vi "Machine Cal UI.vi"() -> ()   [LabVIEW 2013]
uses:
  <vilib>/ptbypt/NI_PtbyPt.lvlib
  <vilib>/Utility/miscctls.llb/LVRowAndColumnTypeDef.ctl
  <vilib>/Analysis/NI_AALPro.lvlib
  Type Defs/Registered Machines.ctl
  <vilib>/Utility/file.llb/Read From Spreadsheet File (string).vi
  <vilib>/event_ctls.llb/lveventtype.ctl
panel:
  in  "View Spreadsheet":bool
  in  "Cal Certificate Path":path
  in  "Cal Cert Started":bool
  in  "Tab.Screen":T1(tab)
  in  "Connection Error":T2(tab)
  in  "Action to Perform":u16(ring) items=["", "Start Calibration", "Continue Calibration", "System Initialization", "System Closeout"]
  in  "IP 4":u8
  in  "IP 3":u8
  in  "IP 2":u8
  in  "IP 1":u8 caption="IP Address"
  in  "pb.sys_connect":bool
  in  "System Type":u16(ring) items=["Continuous Monitoring Tank", "Continuous Module Tank", "Standard Gas Rack", "High-Flow Gas Rack", "Warranty Gas Rack", "Hot Fuel Chamber"]
  in  "Calibration Details":string[][](table)
  in  "Instrument Identification":string[][](table)
  in  "Environment Details":string[][](table)=[["TI Automotive"], ["Caro Test Center"], ["628 Columbia St."], ["Caro, MI 48723"]]
  in  "Standards Used":string[][](table)
  in  "pb.ChanSetup_Forward":bool
  in  "pb.Quit Cal":bool
  in  "Channel Descriptions:":string[][](table)
  in  "Machine Specifications:":string[][](table)
  in  "pb.InfoPage_Back":bool
  in  "pb.SelectionPage_Forward":bool
  in  "pb.ChanSetup_Back":bool
  in  "pb.Cal/Ver_Forward":bool
  in  "Select Units:":enum16{""}(ring)
  out "Tracking":string[][](table)
  in  "Channels Selected:":i32
  in  "pb.Coefficients":bool
  in  "Temperature of room (C)":dbl
  in  "Relative Humidity (%)":dbl
  out "State:":string
  in  "pb.Activate Channels":bool
  in  "Checkbox 12":bool
  in  "pb.Apply 5":bool
  in  "pb.Apply 4":bool
  in  "pb.Apply 3":bool
  in  "pb.Apply 2":bool
  in  "Master Reading":dbl
  in  "Checkbox 2":bool
  in  "Checkbox 1":bool
  out "Units":string
  out "Unit Abbreviation":string
  in  "Channels":string[][](table)=[["", "", "", "", "", "", "", "", "", "", ""]]
  in  "Readings":dbl[](array[numeric])
  in  "pb.Apply 1":bool
  in  "Checkbox 3":bool
  in  "Checkbox 4":bool
  in  "Checkbox 5":bool
  in  "Checkbox 6":bool
  in  "Checkbox 7":bool
  in  "Checkbox 8":bool
  in  "Checkbox 9":bool
  in  "Checkbox 10":bool
  in  "Checkbox 11":bool
  in  "pb.SelectionPage_Back":bool
  in  "[Checkboxes]":T3
  # "*Excel must be closed to return control to this app."
  # "Former Pane: H=499  W=1030"
  # "Tab: H=495  W=1026"
  # "Now thinking it would be better to\nstore that on the RIOs"
  # "Need to have a way to differentiate between a\nnew cal and continuing a cal that is in process"
  # "IP Address"
  # "New System\nCal existing system\nSystem Closeout"
  # "*"
  # "*"
  # "System Not Registered"
  # "*"
  # "*"
  # "*"
  # "*"
  # "System Connection Issue"
  # "*"
  # "*"
  # "*"
  # "*"
  # "RIO Import Issue"
  # "*"
  # "*"
  # "Cannot allow duplicate unit abbreviations or what standard is used to calibrate\na channel is not documented"
  # "Was going to just use a cursive\nfont but dont know if that would\nconstitute a true electronic\nsignature and was not finding\nclear definitions with a quick search"
  # "should be programmatically handled with dropdowns..."
  # "Was thinking I would put expected cal and verify points but I think that\nmight be a problem when it comes to the option of doing multiple\nchannels at once and maybe 1 position used a different cal point"
  # "programmed to the unit abbreviations from channel setup machine specifications"
  # "abbr."
  # "Should always display all and highlight first 4 columns of selected rows"
  # "...have not thought through getting new coefficients would happen"
  # "Incomplete---------------------------------Green\nDone                                                                  Red"
  # "As found\nCalibrate\nVerify"
  # "When I take/retake all readings prompt that new\ncoefficients exist would you like to apply\n\nwould then need a way to store those in case\nthey do not want to apply immediately"
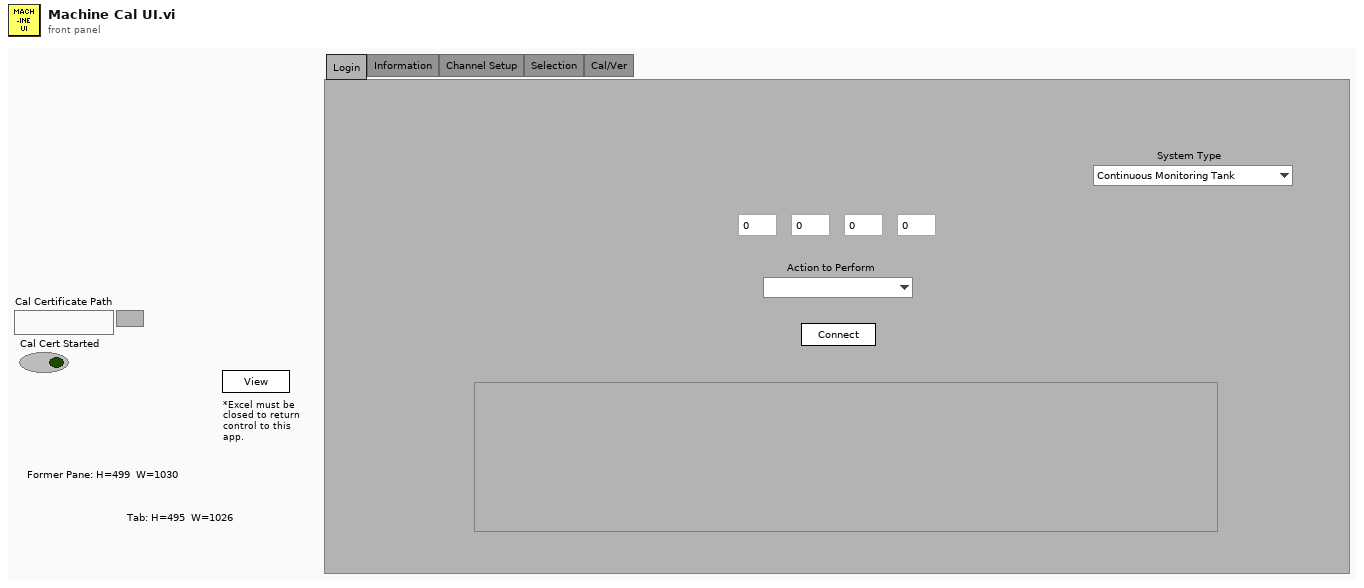
[diagram p1: front panel]
types:
  T1 = enum32{"Login", "Information", "Channel Setup", "Selection", "Cal/Ver"}
  T2 = enum32{"Registration", "Connection", "RIO Import"}
  T3 = cluster{"CB1":bool, "CB2":bool, "CB3":bool, "CB4":bool, "CB5":bool, "CB6":bool, "CB7":bool, "CB8":bool, "CB9":bool, "CB10":bool, "CB11":bool, "CB12":bool}
  T4 = typedef "Registered Machines.ctl" = cluster{"Serial Number":string, "ID":string}
  T5 = cluster{"Certificate Template":path, "Cal Certificate Path":path, "Cal Cert Started":bool, "CalType":u16, "Registered Systems":T4[], "Cal Files Path":path, "Environment Details":string[][], "Instrument Identification":string[][], "Standards Used":string[][], "Calibration Details":string[][], "Machine Specifications:":string[][], "Channel Descriptions:":string[][], "Tracking":string[][], "TrackingRowsSel":i32[], "TrackingTableColors":i32[][], "CalChannelsStorage":string[][], "CalChannelsDisplay":string[][], "ServerStorageFolder":path, "Date FolderPath":path, "Page":enum32{"Login", "Information", "Channel Setup", "Selection", "Cal/Ver"}, "Scroll Flag":bool, "Scroll Check":bool, "Channel Offset":i32, "Checkbox Array":bool[], "Read Array":bool[], "Data Active":bool, "Data Timer":dbl, "Data Timing":dbl, "Full Data":dbl[], "MasterCol":i32, "MasterReading":dbl, "Cal/Ver Data":dbl[], "RIOprogram":string, "IPstring":string, "RIOTempFolder":path, "ServerTempFolder":path, "RoomTemp":dbl, "RelHumidity":dbl, "MaskReadings":bool, "CalState":string, "FoundChannelsStorage":string[][], "VerChannelsStorage":string[][]}
  T6 = enum8{"Enabled", "Disabled", "Disabled and Grayed Out"}
  T7 = enum16{"Init", "Start Data", "Stop Data", "Lost Connection", "Engine Idle", "Write Data", "Read Data"}
  T8 = typedef "lveventtype.ctl" = enum32{"Null", "Timeout", "Annotation Menu Selection", "Annotation Menu Selection?", "App Instance Close", "App Instance Close?", "Autoscale Range Change", "Bookmark Info Change", "Cell Edit", "Cell Edit?", "Cursor Grab", "Cursor Grab?", "Cursor Menu Selection", "Cursor Menu Selection?", "Cursor Move", "Cursor Release", "Data Change", "Direction Change", "Display State Change", "Drag Ended", "Drag Enter", "Drag Leave", "Drag Over", "Drag Source Update", "Drag Starting", "Drag Starting?", "Drop", "Exec State Change", "Key Down", "Key Down?", "Key Repeat", "Key Repeat?", "Key Up", "Listbox Double Click", "Menu Activation?", "Menu Selection (App)", "Menu Selection? (App)", "Menu Selection (User)", "Mouse Down", "Mouse Down?", "Mouse Enter", "Mouse Leave", "Mouse Move", "Mouse Up", "Mouse Wheel", "NI Security User Change (App)", "Pane Size", "Panel Close", "Panel Close?", "Panel Resize", "Plot Attribute Change", "Scale Range Change", "Shortcut Menu Activation?", "Shortcut Menu Selection (App)", "Shortcut Menu Selection? (App)", "Shortcut Menu Selection (User)", "Tree Double Click", "Tree Drag", "Tree Drag?", "Tree Drop", "Tree Drop?", "Tree Item Close", "Tree Item Close?", "Tree Item Open", "Tree Item Open?", "User Event", "Value Change"}
  T9 = typedef "LVRowAndColumnTypeDef.ctl" = cluster{"Row":i32, "Column":i32}
  T10 = typedef "eventvkey.ctl" = enum16{"ASCII", "Enter", "Return", "Shift", "Ctrl", "Alt", "Cmd", "Opt", "Caps", "NumLock", "Clear", "Break", "Up", "Down", "Left", "Right", "Insert", "Delete", "Home", "End", "PageUp", "PageDown", "Escape", "Help", "Pause", "ScrollLock", "F1", "F2", "F3", "F4", "F5", "F6", "F7", "F8", "F9", "F10", "F11", "F12", "F13", "F14", "F15", "F16", "F17", "F18", "F19", "F20", "F21", "F22", "F23", "F24", "Play", "VolumeUp", "VolumeDown", "Mute", "Two Byte Char"}
  T11 = typedef "LVPoint32TypeDef.ctl" = cluster{"Horizontal":i32, "Vertical":i32}
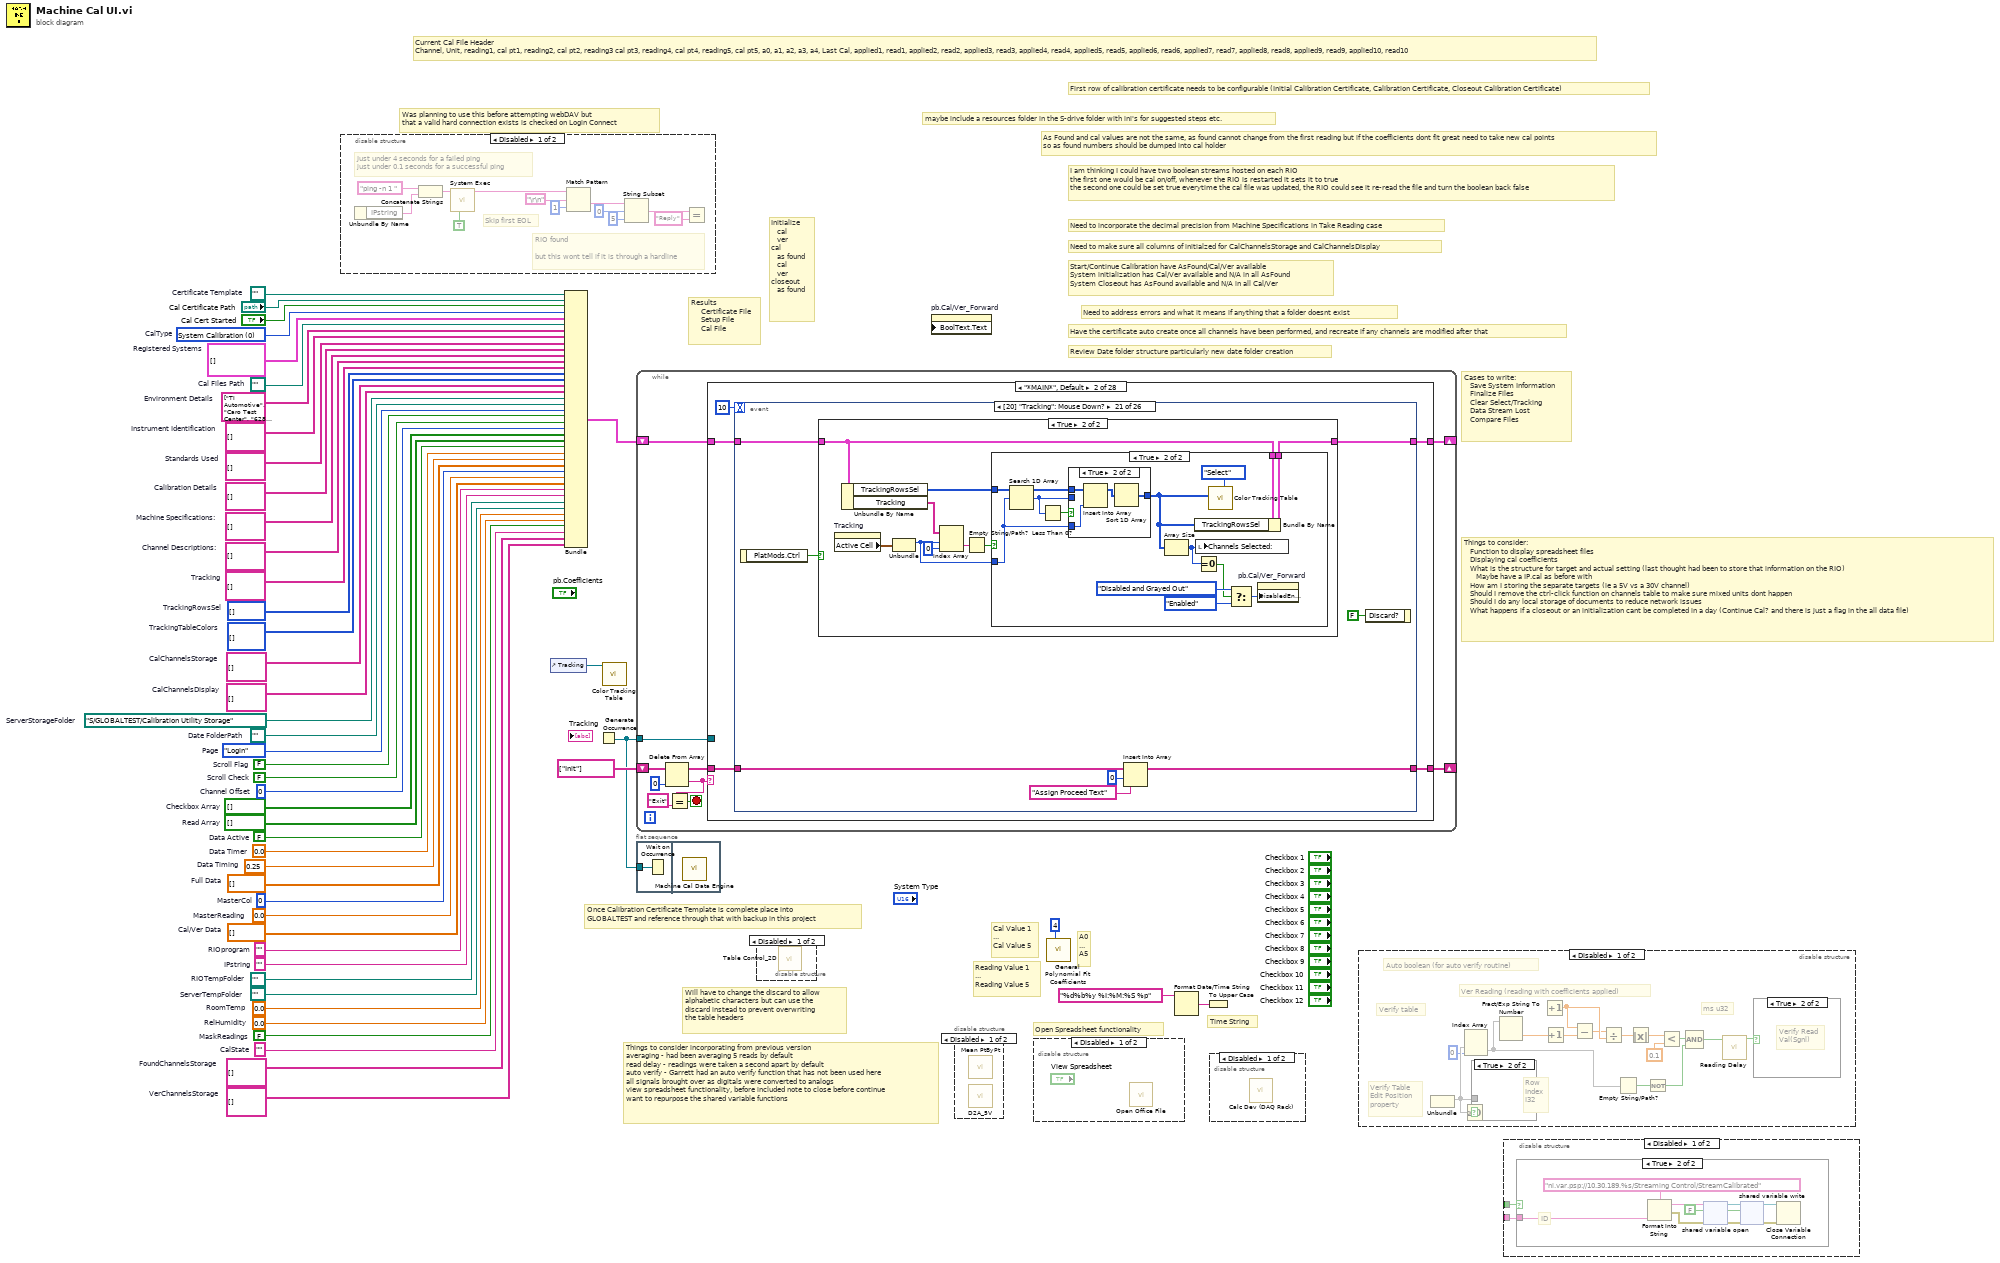
[diagram p0: block diagram]
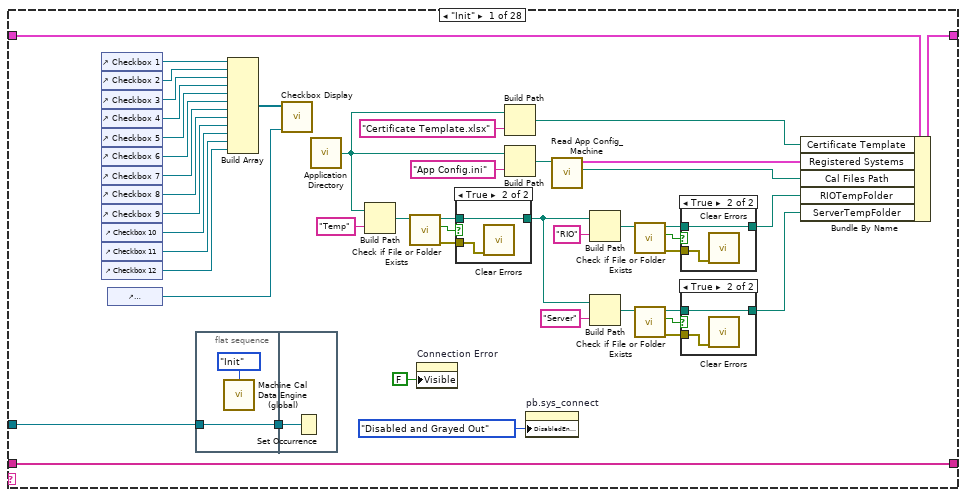
[diagram p12: hidden frame]
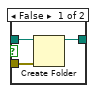
[diagram p13: hidden frame]
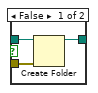
[diagram p14: hidden frame]
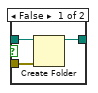
[diagram p15: hidden frame]
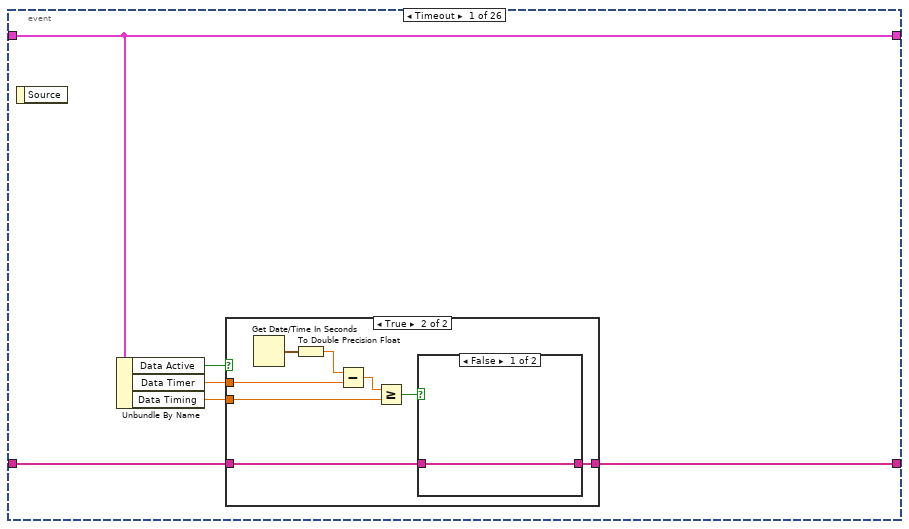
[diagram p16: hidden frame]
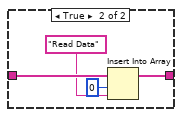
[diagram p18: hidden frame]
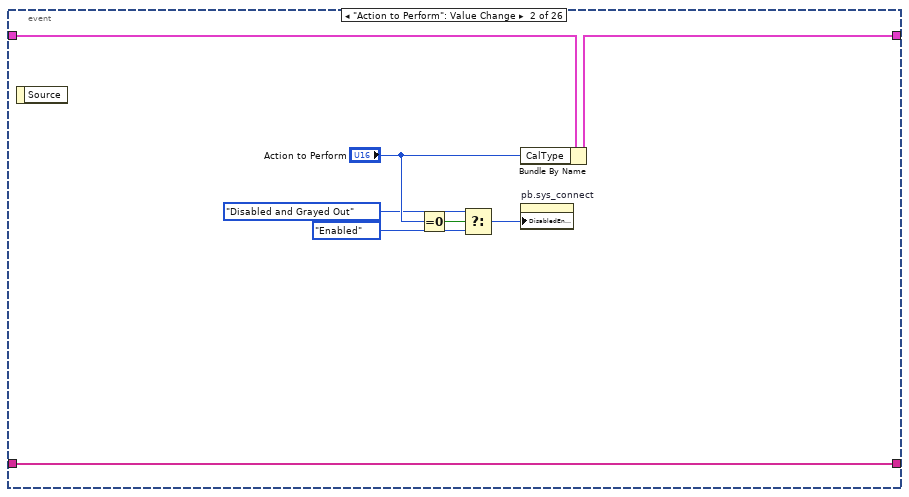
[diagram p19: hidden frame]
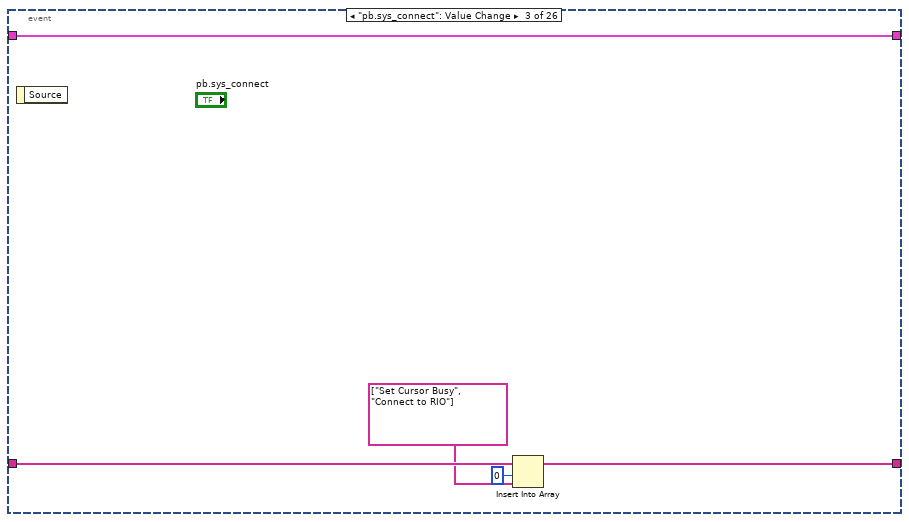
[diagram p20: hidden frame]
diagram:
  w1 = string[][] []  # VerChannelsStorage
  w2 = string[][] []  # FoundChannelsStorage
  w3 = ""  # CalState
  w7 = FALSE  # MaskReadings
  w8 = 0.0  # RelHumidity
  w9 = 0.0  # RoomTemp
  w10 = path ""  # ServerTempFolder
  w11 = path ""  # RIOTempFolder
  w47 = path ""  # Certificate Template
  w12 = ""  # IPstring
  w13 = ""  # RIOprogram
  w15 = dbl[] []  # Cal/Ver Data
  w16 = 0.0  # MasterReading
  w17 = 0  # MasterCol
  w18 = dbl[] []  # Full Data
  w19 = 0.25  # Data Timing
  w20 = 0.0  # Data Timer
  w21 = FALSE  # Data Active
  w22 = bool[] []  # Read Array
  w24 = i32[][] []  # TrackingTableColors
  w25 = i32[] []  # TrackingRowsSel
  w26 = bool[] []  # Checkbox Array
  w27 = 0  # Channel Offset
  w28 = FALSE  # Scroll Check
  w29 = FALSE  # Scroll Flag
  w30 = T1."Login"  # Page
  w31 = string[][] []  # CalChannelsDisplay
  w32 = string[][] []  # CalChannelsStorage
  w33 = path "S:/GLOBALTEST/Calibration Utility Storage"  # ServerStorageFolder
  w34 = path ""  # Date FolderPath
  w35 = string[][] []  # Tracking
  w36 = string[][] []  # Channel Descriptions:
  w37 = string[][] []  # Machine Specifications:
  w38 = string[][] []  # Calibration Details
  w39 = string[][] []  # Standards Used
  w40 = string[][] []  # Instrument Identification
  w41 = string[][] [["TI Automotive"], ["Caro Test Center"], ["628 Columbia St."], ["Caro, MI 48723"], [""], [""], [""]]  # Environment Details
  w43 = T4[] []  # Registered Systems
  w42 = path ""  # Cal Files Path
  w44 = u16 0 items=["System Calibration", "System Initialization", "System Closeout"]  # CalType
  # "Need to address errors and what it means if anything that a folder doesnt exist"
  # "First row of calibration certificate needs to be configurable (Initial Calibration Certificate, Calibration Certificate, Closeout Calibration Certificate)"
  # "As Found and cal values are not the same, as found cannot change from the first reading but if the coefficients dont fit great need to take new cal points\nso as found numbers should be dumped into cal holder"
  # "Time String"
  # "A0\n...\nA5"
  # "Reading Value 1\n...\nReading Value 5"
  # "Cal Value 1\n...\nCal Value 5"
  # "maybe include a resources folder in the S-drive folder with ini's for suggested steps etc."
  # "Things to consider incorporating from previous version\naveraging - had been averaging 5 reads by default\nread delay - readings were taken a second apart by default\nauto verify - Garrett had an auto verify function that has not been used here\nall signals brought over as digitals were converted to analogs\nview spreadsheet functionality, before included note to close before continue\nwant to repurpose the shared variable functions"
  # "Current Cal File Header\nChannel, Unit, reading1, cal pt1, reading2, cal pt2, reading3 cal pt3, reading4, cal pt4, reading5, cal pt5, a0, a1, a2, a3, a4, Last Cal, applied1, read1, applied2, read2, applied3, read3, applied4, read4, applied5, read5, applied6, read6, applied7, read7, applied8, read8, applied9, read9, applied10, read10"
  # "I am thinking I could have two boolean streams hosted on each RIO\nthe first one would be cal on/off, whenever the RIO is restarted it sets it to true\nthe second one could be set true everytime the cal file was updated, the RIO could see it re-read the file and turn the boolean back false"
  # "Was planning to use this before attempting webDAV but\nthat a valid hard connection exists is checked on Login Connect"
  # "Initialize\n   cal\n   ver\ncal\n   as found\n   cal\n   ver\ncloseout\n   as found"
  # "Review Date folder structure particularly new date folder creation"
  # "Have the certificate auto create once all channels have been performed, and recreate if any channels are modified after that"
  # "Things to consider:\n   Function to display spreadsheet files\n   Displaying cal coefficients\n   What is the structure for target and actual setting (last thought had been to store that information on the RIO)\n      Maybe have a IP.cal as before with\n   How am I storing the separate targets (ie a 5V vs a 30V channel)\n   Should I remove the ctrl-click function on channels table to make sure mixed units dont happen\n   Should I do any local storage of documents to reduce network issues\n   What happens if a closeout or an initialization cant be completed in a day (Continue Cal? and there is just a flag in the all data file)"
  # "Open Spreadsheet functionality"
  # "Need to make sure all columns of initialzed for CalChannelsStorage and CalChannelsDisplay"
  # "Need to incorporate the decimal precision from Machine Specifications in Take Reading case"
  # "Start/Continue Calibration have AsFound/Cal/Ver available\nSystem initialization has Cal/Ver available and N/A in all AsFound\nSystem Closeout has AsFound available and N/A in all Cal/Ver"
  # "Cases to write:\n   Save System Information\n   Finalize Files\n   Clear Select/Tracking\n   Data Stream Lost\n   Compare Files"
  # "Results\n     Certificate File\n     Setup File\n     Cal File"
  # "Once Calibration Certificate Template is complete place into\nGLOBALTEST and reference through that with backup in this project"
  # "Will have to change the discard to allow\nalphabetic characters but can use the \ndiscard instead to prevent overwriting\nthe table headers"
  n1 = disable-structure shown="Disabled" {
    frame Disabled {
      # "RIO found\n\nbut this wont tell if it is through a hardline"
      # "Skip first EOL"
      # "Just under 4 seconds for a failed ping\njust under 0.1 seconds for a successful ping"
      n2 = Unbundle By Name() -> ("IPstring"=w52:string)  [unwired: 1 in]
      n3 = Concatenate Strings("ping -n 1 " ("command line"), w52) -> (w50:string)
      n4 = call <vilib>:"System Exec.vi"("run minimized? (F)"=TRUE, "command line"=w50) -> ("standard output"=w54:string)  [unwired: 6 in, 3 out]
      n5 = Match Pattern(string=w54, regular expression="\r\n", offset (0)=1) -> (after substring=w55:string)  [unwired: 3 out]
      n6 = String Subset(string=w55, offset (0)=0, length (rest)=5 ("length (rest)")) -> (substring=w57:string)
      n7 = Equal?(x=w57, y="Reply") -> ()  [unwired: 1 out]
    }
    frame Enabled {
    }
  }
  n8 = control-ref of="Tracking"() -> (w23:refnum<vi>)
  n9 = Bundle("Certificate Template"=w47, "Cal Certificate Path"="Cal Certificate Path", "Cal Cert Started"="Cal Cert Started", "CalType"=w44, "Registered Systems"=w43, "Cal Files Path"=w42, "Environment Details"=w41, "Instrument Identification"=w40, "Standards Used"=w39, "Calibration Details"=w38, "Machine Specifications:"=w37, "Channel Descriptions:"=w36, "Tracking"=w35, "TrackingRowsSel"=w25, "TrackingTableColors"=w24, "CalChannelsStorage"=w32, "CalChannelsDisplay"=w31, "ServerStorageFolder"=w33, "Date FolderPath"=w34, "Page"=w30, "Scroll Flag"=w29, "Scroll Check"=w28, "Channel Offset"=w27, "Checkbox Array"=w26, "Read Array"=w22, "Data Active"=w21, "Data Timer"=w20, "Data Timing"=w19, "Full Data"=w18, "MasterCol"=w17, "MasterReading"=w16, "Cal/Ver Data"=w15, "RIOprogram"=w13, "IPstring"=w12, "RIOTempFolder"=w11, "ServerTempFolder"=w10, "RoomTemp"=w9, "RelHumidity"=w8, "MaskReadings"=w7, "CalState"=w3, "FoundChannelsStorage"=w2, "VerChannelsStorage"=w1) -> (w48:T5)  [unwired: 1 in]
  n10 = Generate Occurrence() -> (w14:refnum<k4>)
  n11 = call "Color Tracking Table.vi"("Tracking Table Ref"=w23) -> ()  [unwired: 11 in]
  n12 = while {
    shift-right: [w65] -> _
    shift-left: string[] ["Init"] -> [w69]
    shift-right: [w63] -> _
    shift-left: w48 -> [w64]
    tunnel: w14 -> [w62]
    stop <- w68 stop-if-true
    n13 = Delete From Array(array=w69, index=0) -> (deleted portion=w67:string, array with subset deleted=w66:string[])  [unwired: 1 in]
    n14 = Equal?(x=w67, y="Exit" ("x")) -> (x = y?=w68:bool)
    n15 = case shown="\"*MAIN*\", Default" w67 {
      selector: w67 -> [_ _ _ _ _ _ _ _ _ _ _ _ _ _ _ _ _ _ _ _ _ _ w829 _ _ w844 _ _]
      tunnel: w66 -> [w117 w139 w442 w464 w469 w496 w523 w534 w589 _ w643 w709 w711 w724 _ _ w741 w747 w753 w786 w814 w817 w824 w832 w834 w845 w857 w870]
      tunnel: [w117 w138 w441 w464 w468 w495 w523 w533 w589 _ w643 w709 w711 w724 _ _ w741 w747 w753 w786 w814 w817 w824 w832 w834 w845 w856 w870] -> w65
      tunnel: w64 -> [w114 w137 w432 w465 w477 w502 w526 w532 w610 _ w642 w688 w714 w733 _ w740 w742 w748 w760 w794 w816 w818 w823 w833 w835 w848 w863 w871]
      tunnel: [w113 w136 w431 w465 w477 w503 w526 w536 w609 _ w641 w687 w713 w732 _ w740 w742 w748 w759 w793 w815 w818 w823 w833 w835 w848 w863 w871] -> w63
      tunnel: w62 -> [w93 _ _ _ _ _ _ _ _ _ _ _ _ _ _ _ _ _ _ _ _ _ _ _ _ _ _ _]
      frame "Init" {
        n16 = control-ref of="Checkbox 1"() -> (w96:refnum<vi>)
        n17 = control-ref of="Checkbox 2"() -> (w97:refnum<vi>)
        n18 = control-ref of="Checkbox 3"() -> (w98:refnum<vi>)
        n19 = control-ref of="Checkbox 4"() -> (w99:refnum<vi>)
        n20 = control-ref of="Checkbox 5"() -> (w100:refnum<vi>)
        n21 = control-ref of="Checkbox 6"() -> (w101:refnum<vi>)
        n22 = control-ref of="Checkbox 7"() -> (w102:refnum<vi>)
        n23 = control-ref of="Checkbox 8"() -> (w103:refnum<vi>)
        n24 = control-ref of="Checkbox 9"() -> (w104:refnum<vi>)
        n25 = control-ref of="Checkbox 10"() -> (w105:refnum<vi>)
        n26 = control-ref of="Checkbox 11"() -> (w106:refnum<vi>)
        n27 = control-ref of="Checkbox 12"() -> (w107:refnum<vi>)
        n28 = control-ref of="[Checkboxes]"() -> (w95:refnum<vi>)
        n29 = flat-sequence {
          tunnel: [w133] -> w94
          tunnel: w93 -> [w133]
          tunnel: w94 -> [w135]
          frame #0 {
            n30 = call "Machine Cal Data Engine (global).vi"("Mode"=T7."Init") -> ()  [unwired: 11 in, 4 out]
          }
          frame #1 {
            n31 = Set Occurrence(w135) -> ()
          }
        }
        n32 = Build Array(w96, w97, w98, w99, w100, w101, w102, w103, w104, w105, w106, w107) -> (w108:refnum<vi>[])
        n33 = call "Checkbox Display.vi"("[Checkboxes] Ref"=w95, "Checkbox Refs"=w108) -> ()  [unwired: 10 in]
        n34 = call <vilib>:"Application Directory.vi"() -> ("Application Directory"=w90:path)
        n35 = Build Path(base path=w90, name or relative path="Temp") -> (appended path=w88:path)
        n36 = call <vilib>:"Check if File or Folder Exists.vi"("path"=w88) -> ("error out"=w85:errorcluster, "file or folder exists?"=w87:bool, "dup path"=w86:path)  [unwired: 8 in]
        n37 = property on="Connection Error" class="TabCtl (strict)"("Visible"=FALSE) -> ()  [unwired: 2 in, 2 out]
        n38 = case shown="True" w87 {
          tunnel: w86 -> [w130 w132]
          tunnel: w85 -> [w128 w131]
          tunnel: [w129 w132] -> w74
          frame False {
            n39 = Create Folder(path (use dialog)=w130, error in=w128) -> (created path=w129:path)  [unwired: 1 in, 2 out]
          }
          frame True {
            n40 = call <vilib>:"Clear Errors.vi"("error in (no error)"=w131) -> ()  [unwired: 6 in, 1 out]
          }
        }
        n41 = Build Path(base path=w90, name or relative path="Certificate Template.xlsx") -> (appended path=w91:path)
        n42 = Build Path(base path=w90, name or relative path="App Config.ini") -> (appended path=w116:path)
        n43 = property on="pb.sys_connect" class="Bool"("DisabledEnum"=T6."Disabled and Grayed Out" ("Disabled")) -> ()  [unwired: 2 in, 2 out]
        n44 = call "Read App Config_Machine.vi"("App Config Path"=w116) -> ("Cal Files Path"=w111:path, "Registered Systems"=w112:T4[])  [unwired: 9 in]
        n45 = Build Path(base path=w74, name or relative path="RIO") -> (appended path=w83:path)
        n46 = Build Path(base path=w74, name or relative path="Server") -> (appended path=w76:path)
        n47 = call <vilib>:"Check if File or Folder Exists.vi"("path"=w83) -> ("error out"=w80:errorcluster, "file or folder exists?"=w82:bool, "dup path"=w81:path)  [unwired: 8 in]
        n48 = call <vilib>:"Check if File or Folder Exists.vi"("path"=w76) -> ("error out"=w79:errorcluster, "file or folder exists?"=w77:bool, "dup path"=w78:path)  [unwired: 8 in]
        n49 = case shown="True" w82 {
          tunnel: w81 -> [w125 w127]
          tunnel: w80 -> [w123 w126]
          tunnel: [w124 w127] -> w73
          frame False {
            n50 = Create Folder(path (use dialog)=w125, error in=w123) -> (created path=w124:path)  [unwired: 1 in, 2 out]
          }
          frame True {
            n51 = call <vilib>:"Clear Errors.vi"("error in (no error)"=w126) -> ()  [unwired: 6 in, 1 out]
          }
        }
        n52 = case shown="True" w77 {
          tunnel: w78 -> [w120 w122]
          tunnel: w79 -> [w118 w121]
          tunnel: [w119 w122] -> w72
          frame False {
            n53 = Create Folder(path (use dialog)=w120, error in=w118) -> (created path=w119:path)  [unwired: 1 in, 2 out]
          }
          frame True {
            n54 = call <vilib>:"Clear Errors.vi"("error in (no error)"=w121) -> ()  [unwired: 6 in, 1 out]
          }
        }
        n55 = Bundle By Name(cluster=w114, "Certificate Template"=w91, "Registered Systems"=w112, "Cal Files Path"=w111, "RIOTempFolder"=w73, "ServerTempFolder"=w72) -> (w113:T5)
      }
      frame "*MAIN*", Default {
        n56 = event shown="[20] \"Tracking\": Mouse Down?" {
          selector: _ -> [_ _ _ _ _ _ _ _ _ _ _ _ _ _ _ _ _ _ _ _ _ _ _ _ _ _]
          dyn-events: _ -> [_ _ _ _ _ _ _ _ _ _ _ _ _ _ _ _ _ _ _ _ _ _ _ _ _ _]
          timeout: 10 -> [_ _ _ _ _ _ _ _ _ _ _ _ _ _ _ _ _ _ _ _ _ _ _ _ _ _]
          tunnel: w139 -> [w145 w166 w172 w176 w181 w186 w190 w195 w201 w206 w209 w234 w238 w242 w246 w251 w254 w260 w278 w292 w320 w358 w380 w409 w421 w425]
          tunnel: [w144 w166 w171 w175 w180 w185 w191 w196 w200 w205 w209 w234 w238 w242 w246 w251 w254 w260 w277 w290 w319 w358 w380 w408 w421 w425] -> w138
          tunnel: w137 -> [w146 w168 w169 w174 w179 w184 w189 w194 w199 w204 w210 w237 w241 w245 w249 w253 w257 w259 w279 w300 w324 w362 w382 w412 w424 w429]
          tunnel: [w146 w167 w169 w174 w179 w184 w189 w194 w199 w204 w210 w236 w240 w244 w247 w252 w256 w261 w279 w299 w323 w361 w381 w411 w423 w428] -> w136
          event Timeout {
            n57 = event-data() -> ()  [unwired: 1 in, 1 out]
            n58 = Unbundle By Name(w146) -> ("Data Active"=w143:bool, "Data Timer"=w142:dbl, "Data Timing"=w141:dbl)
            n59 = case shown="True" w143 {
              tunnel: w145 -> [w147 w155]
              tunnel: [w147 w154] -> w144
              tunnel: w142 -> [_ w149]
              tunnel: w141 -> [_ w150]
              frame False {
              }
              frame True {
                n60 = Get Date/Time In Seconds() -> (seconds since 1Jan1904=w153:timestamp)
                n61 = To Double Precision Float(number=w153) -> (double precision float=w152:dbl)
                n62 = Subtract(x=w152, y=w149) -> (x-y=w151:dbl)
                n63 = Greater Or Equal?(x=w151, y=w150) -> (x >= y?=w148:bool)
                n64 = case shown="False" w148 {
                  tunnel: w155 -> [w156 w160]
                  tunnel: [w156 w159] -> w154
                  frame False {
                  }
                  frame True {
                    n65 = Insert Into Array(array=w160, index=0, new element="Read Data") -> (w159:string[])
                  }
                }
              }
            }
          }
          event "Action to Perform": Value Change {
            n66 = event-data() -> ()  [unwired: 1 in, 1 out]
            n67 = Equal To 0?(x="Action to Perform") -> (x = 0?=w164:bool)
            n68 = Select(t=T6."Disabled and Grayed Out" ("Disabled"), s=w164, f=T6."Enabled" ("Disabled")) -> (s? t:f=w162:T6)
            n69 = Bundle By Name(cluster=w168, "CalType"="Action to Perform") -> (w167:T5)
            n70 = property on="pb.sys_connect" class="Bool"("DisabledEnum"=w162) -> ()  [unwired: 2 in, 2 out]
          }
          event "pb.sys_connect": Value Change {
            n71 = event-data() -> ()  [unwired: 1 in, 1 out]
            n72 = Insert Into Array(array=w172, index=0, new element=string[] ["Set Cursor Busy", "Connect to RIO"]) -> (w171:string[])
          }
          event "pb.Quit Cal": Value Change {
            n73 = event-data() -> ()  [unwired: 1 in, 1 out]
            n74 = Insert Into Array(array=w176, index=0, new element=string[] ["Save System Information", "Return to Login"]) -> (w175:string[])
          }
          event "pb.ChanSetup_Forward": Value Change {
            n75 = event-data() -> ()  [unwired: 1 in, 1 out]
            n76 = Insert Into Array(array=w181, index=0, new element=string[] ["Save System Information", "Display Chan Setup Tab"]) -> (w180:string[])
          }
          event "pb.InfoPage_Back": Value Change {
            n77 = event-data() -> ()  [unwired: 1 in, 1 out]
            n78 = Insert Into Array(array=w186, index=0, new element=string[] ["Save Chan Setup", "Display Info Tab"]) -> (w185:string[])
          }
          event "pb.SelectionPage_Forward": Value Change {
            n79 = event-data() -> ()  [unwired: 1 in, 1 out]
            n80 = Insert Into Array(array=w190, index=0, new element=string[] ["Save Chan Setup", "Display Selection Tab"]) -> (w191:string[])
          }
          event "pb.ChanSetup_Back": Value Change {
            n81 = event-data() -> ()  [unwired: 1 in, 1 out]
            n82 = Insert Into Array(array=w195, index=0, new element=string[] ["Display Chan Setup Tab"]) -> (w196:string[])
          }
          event "pb.Cal/Ver_Forward": Value Change {
            n83 = event-data() -> ()  [unwired: 1 in, 1 out]
            n84 = Insert Into Array(array=w201, index=0, new element=string[] ["Display Cal/Ver Tab"]) -> (w200:string[])
          }
          event "pb.SelectionPage_Back": Value Change {
            n85 = event-data() -> ()  [unwired: 1 in, 1 out]
            n86 = Insert Into Array(array=w206, index=0, new element=string[] ["Cancel Cal/Ver", "Display Selection Tab"]) -> (w205:string[])
          }
          event "IP 1", "IP 2", "IP 3", "IP 4": Key Down? {
            n87 = event-data() -> ("Char"=w221:i16, "CtlRef"=w214:refnum<vi>, "VKey"=w223:T10, "ScanCode"=w222:i16)  [unwired: 1 in]
            n88 = control-ref of="IP 1"() -> (w217:refnum<vi>)
            n89 = control-ref of="IP 2"() -> (w219:refnum<vi>)
            n90 = control-ref of="IP 3"() -> (w216:refnum<vi>)
            n91 = control-ref of="IP 4"() -> (w215:refnum<vi>)
            n92 = control-ref of="System Type"() -> (w218:refnum<vi>)
            n93 = Build Array(w217, w219, w216, w215) -> (w213:refnum<vi>[])
            n94 = Build Array(w219, w216, w215, w218) -> (w212:refnum<vi>[])
            n95 = for {
              tunnel: w214 -> [w227]
              tunnel: w213 -> [w226] mode=indexing
              tunnel: w212 -> [w224] mode=indexing
              tunnel: [w224] -> w211
              stop <- w225 stop-if-true
              n96 = Equal?(x=w227, y=w226) -> (x = y?=w225:bool)
            }
            n97 = case shown="\"Enter\", \"Return\", \"Right\"" w223 {
              tunnel: [w232 TRUE] -> w220
              tunnel: w222 -> [w231 _]
              frame "ASCII", Default {
                n98 = Equal?(x=i16 15, y=w231) -> (x = y?=w232:bool)
              }
              frame "Enter", "Return", "Right" {
              }
            }
            n99 = case shown="True" w220 {
              tunnel: w211 -> [_ w228]
              frame False {
              }
              frame True {
                n100 = property class="Num"(reference=w228, "Key Focus"=TRUE) -> ()  [unwired: 1 in, 2 out]
              }
            }
            n101 = event-data("Char"=w221) -> ()  [unwired: 1 in, 1 out]
          }
          event "Environment Details": Value Change {
            n102 = event-data() -> ()  [unwired: 1 in, 1 out]
            n103 = Bundle By Name(cluster=w237, "Environment Details"="Environment Details") -> (w236:T5)
          }
          event "Instrument Identification": Value Change {
            n104 = event-data() -> ()  [unwired: 1 in, 1 out]
            n105 = Bundle By Name(cluster=w241, "Instrument Identification"="Instrument Identification") -> (w240:T5)
          }
          event "Standards Used": Value Change {
            n106 = event-data() -> ()  [unwired: 1 in, 1 out]
            n107 = Bundle By Name(cluster=w245, "Standards Used"="Standards Used") -> (w244:T5)
          }
          event "Calibration Details": Value Change {
            n108 = event-data() -> ()  [unwired: 1 in, 1 out]
            n109 = Bundle By Name(cluster=w249, "Calibration Details"="Calibration Details") -> (w247:T5)
          }
          event "Machine Specifications:": Value Change {
            n110 = event-data() -> ()  [unwired: 1 in, 1 out]
            n111 = Bundle By Name(cluster=w253, "Machine Specifications:"="Machine Specifications:") -> (w252:T5)
          }
          event "Channel Descriptions:": Value Change {
            n112 = event-data() -> ()  [unwired: 1 in, 1 out]
            n113 = Bundle By Name(cluster=w257, "Channel Descriptions:"="Channel Descriptions:") -> (w256:T5)
          }
          event "Channels": Mouse Down {
            n114 = event-data() -> ("Coords"=w262:T11)  [unwired: 1 in]
            n115 = Unbundle By Name(w259) -> ("Scroll Check"=w258:bool)
            n116 = case shown="True" w258 {
              tunnel: w262 -> [_ w273]
              tunnel: [w264 w268] -> w261
              tunnel: w259 -> [w265 w266]
              frame False {
                # "12 or fewer channels, no scroll bar"
                n117 = Bundle By Name(cluster=w265, "Scroll Flag"=FALSE) -> (w264:T5)
              }
              frame True {
                # "More than 12 channels, check if mouse was on scroll bar"
                # "Set Scroll Flag"
                # "Width:\n787 - No scrollbar\n804 - Yes scrollbar"
                # "Make it table referenced"
                n118 = Unbundle By Name(w273) -> ("Horizontal"=w272:i32)
                n119 = property on="Channels" class="Tbl (strict)"() -> ("Left"=w271:i32)  [unwired: 2 in, 2 out]
                n120 = Subtract(x=w272, y=w271) -> (x-y=w270:i32)
                n121 = Greater Or Equal?(x=w270, y=787) -> (x >= y?=w267:bool)
                n122 = Bundle By Name(cluster=w266, "Scroll Flag"=w267) -> (w268:T5)
              }
            }
          }
          event "Channels": Mouse Up; "Channels": Mouse Wheel {
            n123 = event-data() -> ("Type"=w283:T8)  [unwired: 1 in]
            n124 = Unbundle By Name(w279) -> ("Scroll Check"=w276:bool, "Scroll Flag"=w280:bool)
            n125 = Equal?(x=w283, y=lveventtype."Mouse Wheel" ("Type")) -> (x = y?=w281:bool)
            n126 = Or(x=w280, y=w281) -> (x .or. y?=w275:bool)
            n127 = And(x=w276, y=w275) -> (x .and. y?=w274:bool)
            n128 = case shown="True" w274 {
              tunnel: w278 -> [w284 w286]
              tunnel: [w284 w285] -> w277
              frame False {
              }
              frame True {
                n129 = Insert Into Array(array=w286, index=0, new element=string[] ["Scroll Channels"]) -> (w285:string[])
              }
            }
          }
          event "Select Units:": Value Change {
            n130 = event-data() -> ()  [unwired: 1 in, 1 out]
            n131 = Unbundle By Name(w300) -> ("Tracking"=w304:string[][])
            n132 = Equal To 0?(x="Select Units:") -> (x = 0?=w301:bool)
            n133 = case shown="False" w301 {
              tunnel: w304 -> [_ w313]
              tunnel: "Select Units:" -> [_ w309]
              tunnel: [i32[] [] w308] -> w298
              tunnel: [0 w307] -> w297
              frame True {
                # "No channels selected"
              }
              frame False {
                n134 = property on="Select Units:" class="Enum (strict)"() -> ("Strings []"=w314:string[])  [unwired: 2 in, 2 out]
                n135 = Index Array(array=w313, index (col)=2 ("disabled index (col)")) -> (element=w311:string[])  [unwired: 1 in]
                n136 = Index Array(array=w314, index=w309) -> (element=w310:string)
                n137 = for {
                  tunnel: w311 -> [w318] mode=indexing
                  tunnel: w310 -> [w317]
                  tunnel: [w316] -> w308 mode=indexing if=w315
                  i -> [w316]
                  n138 = Equal?(x=w318, y=w317) -> (x = y?=w315:bool)
                }
                n139 = Array Size(array=w308) -> (size(s)=w307:i32)
              }
            }
            n140 = Insert Into Array(array=w292, index=0, new element="Assign Proceed Text" ("new element/subarray")) -> (w290:string[])
            n141 = Equal To 0?(x=w297) -> (x = 0?=w293:bool)
            n142 = call "Color Tracking Table.vi"("Mode"=enum16{"Select", "Track"}."Select", "TrackingRowsSelected"=w298) -> ()  [unwired: 10 in]
            n143 = Bundle By Name(cluster=w300, "TrackingRowsSel"=w298) -> (w299:T5)
            n144 = local write "Channels Selected:"(w297) -> ()
            n145 = Select(t=T6."Disabled and Grayed Out" ("Disabled"), s=w293, f=T6."Enabled" ("Disabled")) -> (s? t:f=w294:T6)
            n146 = property on="pb.Cal/Ver_Forward" class="Bool"("DisabledEnum"=w294) -> ()  [unwired: 2 in, 2 out]
          }
          event "Tracking": Mouse Down? {
            n147 = event-data() -> ("PlatMods.Ctrl"=w325:bool)  [unwired: 1 in]
            n148 = case shown="True" w325 {
              tunnel: w324 -> [w327 w334]
              tunnel: [w327 w336] -> w323
              frame False {
              }
              frame True {
                n149 = property on="Tracking" class="Tbl (strict)"() -> ("Active Cell"=w335:T9)  [unwired: 2 in, 2 out]
                n150 = Unbundle By Name(w334) -> ("TrackingRowsSel"=w329:i32[], "Tracking"=w333:string[][])
                n151 = Unbundle(w335) -> ("Row"=w328:i32)  [unwired: 1 out]
                n152 = Index Array(array=w333, index (row)=w328, index (col)=0 ("disabled index (col)")) -> (element=w331:string)
                n153 = Empty String/Path?(string/path=w331) -> (empty?=w330:bool)
                n154 = case shown="True" w330 {
                  tunnel: [w337 w350] -> w336
                  tunnel: w334 -> [w337 w349]
                  tunnel: w329 -> [_ w341]
                  tunnel: w328 -> [_ w340]
                  frame False {
                  }
                  frame True {
                    n155 = Search 1D Array(1D array=w341, element=w340) -> (index of element=w339:i32)  [unwired: 1 in]
                    n156 = Less Than 0?(x=w339) -> (x < 0?=w342:bool)
                    n157 = case shown="True" w342 {
                      tunnel: w341 -> [w353 w357]
                      tunnel: [w351 w355] -> w338
                      tunnel: w340 -> [_ w354]
                      tunnel: w339 -> [w352 _]
                      frame False {
                        n158 = Delete From Array(array=w353, index=w352) -> (array with subset deleted=w351:i32[])  [unwired: 1 in, 1 out]
                      }
                      frame True {
                        n159 = Insert Into Array(array=w357, new element=w354) -> (w356:i32[])  [unwired: 1 in]
                        n160 = Sort 1D Array(array=w356) -> (sorted array=w355:i32[])
                      }
                    }
                    n161 = Array Size(array=w338) -> (size(s)=w343:i32)
                    n162 = Bundle By Name(cluster=w349, "TrackingRowsSel"=w338) -> (w350:T5)
                    n163 = local write "Channels Selected:"(w343) -> ()
                    n164 = Equal To 0?(x=w343) -> (x = 0?=w344:bool)
                    n165 = call "Color Tracking Table.vi"("Mode"=enum16{"Select", "Track"}."Select", "TrackingRowsSelected"=w338) -> ()  [unwired: 10 in]
                    n166 = Select(t=T6."Disabled and Grayed Out" ("Disabled"), s=w344, f=T6."Enabled" ("Disabled")) -> (s? t:f=w345:T6)
                    n167 = property on="pb.Cal/Ver_Forward" class="Bool"("DisabledEnum"=w345) -> ()  [unwired: 2 in, 2 out]
                  }
                }
              }
            }
            n168 = Insert Into Array(array=w320, index=0, new element="Assign Proceed Text" ("new element/subarray")) -> (w319:string[])
            n169 = event-data("Discard?"=FALSE) -> ()  [unwired: 1 in, 1 out]
          }
          event "[Checkboxes]": Value Change {
            n170 = event-data() -> ()  [unwired: 1 in, 1 out]
            n171 = Unbundle By Name(w362) -> ("Scroll Check"=w364:bool, "Checkbox Array"=w360:bool[], "Channel Offset"=w359:i32)
            n172 = case shown="False" w364 {
              tunnel: "[Checkboxes]" -> [w371 w372]
              tunnel: w362 -> [w370 w377]
              tunnel: [w369 w376] -> w361
              tunnel: w360 -> [w368 w378]
              tunnel: w359 -> [_ w373]
              frame False {
                # "Used to keep correct amount of entries"
                # "12 or less channels no checks"
                n173 = Cluster To Array(cluster=w371) -> (array=w366:bool[])
                n174 = Replace Array Subset(array=w368, new element=w366, index=0) -> (w365:bool[])
                n175 = Bundle By Name(cluster=w370, "Checkbox Array"=w365) -> (w369:T5)
              }
              frame True {
                # "Was worried if I have 12 channels from [Checkboxes] but less than 12 are displayed\nfrom scrolling that the array would become larger but checked that does not happen"
                # "More than 12 channels, look at where we are in the table"
                n176 = Cluster To Array(cluster=w372) -> (array=w375:bool[])
                n177 = Replace Array Subset(array=w378, new element=w375, index=w373) -> (w374:bool[])
                n178 = Bundle By Name(cluster=w377, "Checkbox Array"=w374) -> (w376:T5)
              }
            }
          }
          event "pb.Activate Channels": Value Change {
            n179 = event-data() -> ()  [unwired: 1 in, 1 out]
            n180 = case shown="True" "pb.Activate Channels" {
              tunnel: w382 -> [w384 w393]
              tunnel: [w384 w392] -> w381
              frame False {
                # "Stop reading on engine"
                n181 = call "Machine Cal Data Engine (global).vi"("Mode"=T7."Stop Data") -> ()  [unwired: 11 in, 4 out]
              }
              frame True {
                # "Will the repeat initialize cause a memory issue?"
                # "Activate reading in engine"
                n182 = Unbundle By Name(w393) -> ("TrackingRowsSel"=w395:i32[], "Checkbox Array"=w394:bool[], "Tracking"=w391:string[][])
                n183 = for {
                  tunnel: w395 -> [w405] mode=indexing
                  tunnel: [w405] -> w386 mode=indexing if=w404
                  tunnel: w394 -> [w404] mode=indexing
                }
                n184 = Array Size(array=w391) -> (size(s)=w390:i32[])
                n185 = Index Array(array=w390) -> (element=w389:i32)  [unwired: 1 in]
                n186 = Initialize Array(FALSE, w389) -> (w387:bool[])
                n187 = for {
                  shift-right: [w402] -> w385
                  shift-left: w387 -> [w403]
                  tunnel: w386 -> [w401] mode=indexing
                  n188 = Replace Array Subset(array=w403, new element=TRUE, index=w401) -> (w402:bool[])
                }
                n189 = flat-sequence {
                  tunnel: w393 -> [w398]
                  tunnel: [w397] -> w392
                  tunnel: w385 -> [w396]
                  frame #0 {
                    n190 = Bundle By Name(cluster=w398, "Read Array"=w396) -> (w397:T5)
                    n191 = call "Machine Cal Data Engine (global).vi"("Mode"=T7."Start Data") -> ()  [unwired: 11 in, 4 out]
                  }
                }
              }
            }
          }
          event "pb.Apply 1", "pb.Apply 2", "pb.Apply 3", "pb.Apply 4", "pb.Apply 5": Value Change {
            n192 = event-data() -> ("CtlRef"=w414:refnum<vi>)  [unwired: 1 in]
            n193 = property class="Bool"(reference=w414) -> ("Label.Text"=w413:string)  [unwired: 1 in, 2 out]
            n194 = case shown="\"pb.Apply 3\"" w413 {
              tunnel: [1 ("index") 3 ("index") 5 ("index") 7 ("index") 9 ("index")] -> w410
              frame "pb.Apply 1", Default {
              }
              frame "pb.Apply 2" {
              }
              frame "pb.Apply 3" {
              }
              frame "pb.Apply 4" {
              }
              frame "pb.Apply 5" {
              }
            }
            n195 = Insert Into Array(array=w409, index=0, new element="Take Reading" ("new element/subarray")) -> (w408:string[])
            n196 = Bundle By Name(cluster=w412, "MasterCol"=w410) -> (w411:T5)
          }
          event "Master Reading": Value Change {
            n197 = event-data() -> ()  [unwired: 1 in, 1 out]
            n198 = Not A Number/Path/Refnum?(number/path/refnum="Master Reading") -> (NaN/Path/Refnum?=w420:bool)
            n199 = Bundle By Name(cluster=w424, "MasterReading"="Master Reading", "MaskReadings"=w420) -> (w423:T5)
          }
          event "Temperature of room (C)", "Relative Humidity (%)": Value Change {
            n200 = event-data() -> ()  [unwired: 1 in, 1 out]
            n201 = Bundle By Name(cluster=w429, "RoomTemp"="Temperature of room (C)", "RelHumidity"="Relative Humidity (%)") -> (w428:T5)
          }
        }
      }
      frame "Connect to RIO" {
        # "Cal Types:\n   0-Blank (locked out)\n   1-Start Calibration\n   2-Continue Calibration\n   3-System Initialization\n   4-System Closeout"
        # "cDAQs don't have the same IP base"
        n202 = Format Into String(format string="%g.%g.%g.%g", "IP 1", "IP 2", "IP 3", "IP 4") -> (resulting string=w430:string)  [unwired: 2 in, 1 out]
        n203 = Unbundle By Name(w432) -> ("CalType"=w438:u16, "Registered Systems"=w445:T4[])
        n204 = for {
          tunnel: w445 -> [w461] mode=indexing
          tunnel: w430 -> [w459]
          tunnel: [w458] -> w444
          tunnel: [w457] -> w434
          stop <- w457 stop-if-true
          n205 = Unbundle(w461) -> ("Serial Number"=w458:string, "ID"=w460:string)
          n206 = Equal?(x=w460, y=w459) -> (x = y?=w457:bool)
        }
        n207 = case shown="1, 4" w438 {
          tunnel: [string[] ["Setup WebDAV", "Import From RIO", "Load Info/Channels", "Create Date Folder", "Clear Select/Tracking", "Display Info Tab", "Unset Cursor Busy"] string[] ["Setup WebDAV", "Import From RIO", "Load Info/Channels", "Load Select/Tracking", "Display Info Tab", "Unset Cursor Busy"] string[] ["Setup WebDAV", "Create Date Folder", "Clear Info/Channels", "Clear Select/Tracking", "Display Info Tab", "Unset Cursor Busy"] string[] ["Unset Cursor Busy"]] -> w437
          frame 1, 4 {
            # "System Closeout"
            # "Start Calibration"
          }
          frame 2 {
            # "Continue Calibration"
          }
          frame 3 {
            # "System Initialization"
          }
          frame 0, Default {
            n208 = One Button Dialog(message="No action selected\n\nReport to programmer") -> ()  [unwired: 1 in, 1 out]
          }
        }
        n209 = call "Find Network Systems.vi"() -> ("Serial Number"=w446:string)  [unwired: 10 in, 1 out]
        n210 = Equal?(x=w446, y=w444) -> (x = y?=w440:bool)
        n211 = Bundle By Name(cluster=w432, "IPstring"=w430) -> (w431:T5)
        n212 = Select(t=string[] ["System Not Found", "Unset Cursor Busy"], s=w434, f=string[] ["System Not Registered", "Unset Cursor Busy"]) -> (s? t:f=w433:string[])
        n213 = Select(t=w437, s=w440, f=w433) -> (s? t:f=w439:string[])
        n214 = Insert Into Array(array=w442, index=0, new element=w439) -> (w441:string[])
      }
      frame "Setup WebDAV" {
        n215 = Unbundle By Name(w465) -> ("IPstring"=w463:string)
        n216 = call "WebDAV transfer.vi"("IPstring"=w463, "Mode"=enum16{"Setup", "Retrieve File", "Export File"}."Setup") -> ()  [unwired: 13 in, 1 out]
      }
      frame "Import From RIO" {
        # "Only comes to this case if it is a:\n   Start Calibration\n   Continue Calibration\n   System Closeout"
        n217 = Unbundle By Name(w477) -> ("RIOTempFolder"=w474:path)
        n218 = local read "IP 4"() -> (w475:u8)
        n219 = Format Into String(format string="%g.cal", w475) -> (resulting string=w473:string)  [unwired: 2 in, 1 out]
        n220 = flat-sequence {
          tunnel: [w488] -> w472
          tunnel: w474 -> [w488]
          tunnel: w473 -> [w489]
          tunnel: [w487] -> w467
          tunnel: w472 -> [w492]
          tunnel: [w491] -> w471
          frame #0 {
            n221 = call "WebDAV transfer.vi"("Mode"=enum16{"Setup", "Retrieve File", "Export File"}."Retrieve File", "Local Folder"=w488, "Filename"=w489) -> ("Error Out"=w487:errorcluster)  [unwired: 12 in]
          }
          frame #1 {
            n222 = call "WebDAV transfer.vi"("Mode"=enum16{"Setup", "Retrieve File", "Export File"}."Retrieve File", "Local Folder"=w492, "Filename"="Setup.info") -> ("Error Out"=w491:errorcluster)  [unwired: 12 in]
          }
        }
        n223 = Unbundle By Name(w467) -> ("status"=w466:bool)
        n224 = Unbundle By Name(w471) -> ("status"=w470:bool)
        n225 = case shown="True" w466 {
          tunnel: w470 -> [_ w481]
          tunnel: w469 -> [_ w480]
          tunnel: [string[] ["RIO Import Error"] w479] -> w468
          frame True {
          }
          frame False {
            n226 = case shown="False" w481 {
              tunnel: w480 -> [w485 w486]
              tunnel: [w484 w486] -> w479
              frame False {
                # "Load files from server"
                # "Had been done with\nnew cal utility"
                # "No Error - File loaded"
                n227 = Insert Into Array(array=w485, index=0, new element="Import From Server" ("new element/subarray")) -> (w484:string[])
              }
              frame True {
                # "no action"
                # "Assuming this is the first time\ndone with new cal utility"
                # "Error"
              }
            }
          }
        }
      }
      frame "Import From Server" {
        # "The only time an IP folder is created is if there\nis if the folders below them are being created"
        # "could I have a closeout\nrio gets reassigned to new system\nand new cal all start within the same day"
        # "(needs to be only folder)"
        # "Find first folder (gauge #)"
        # "Find most recent\ndate_program folder"
        n228 = local read "IP 1"() -> (w513:u8)
        n229 = local read "IP 2"() -> (w514:u8)
        n230 = local read "IP 3"() -> (w515:u8)
        n231 = local read "IP 4"() -> (w516:u8)
        n232 = Unbundle By Name(w502) -> ("ServerStorageFolder"=w517:path)  [unwired: 1 out]
        n233 = Format Into String(format string="%g_%g_%g_%g", initial string="Storage\\", w513, w514, w515, w516) -> (resulting string=w511:string)  [unwired: 1 in, 1 out]
        n234 = Build Path(base path=w517, name or relative path=w511) -> (appended path=w500:path)
        n235 = call <vilib>:"Check if File or Folder Exists.vi"("path"=w500) -> ("dup path"=w499:path)  [unwired: 8 in, 2 out]
        n236 = List Folder(path=w499) -> (folder names=w509:string[])  [unwired: 3 in, 3 out]
        n237 = Sort 1D Array(array=w509) -> (sorted array=w510:string[])
        n238 = Delete From Array(array=w510) -> (deleted portion=w508:string)  [unwired: 2 in, 1 out]
        n239 = Build Path(base path=w499, name or relative path=w508) -> (appended path=w507:path)
        n240 = Insert Into Array(array=w496, index=0, new element="Compare Files" ("new element/subarray")) -> (w495:string[])
        n241 = List Folder(path=w507) -> (folder names=w506:string[])  [unwired: 3 in, 3 out]
        n242 = Index Array(array=w506) -> (element=w505:string)  [unwired: 1 in]
        n243 = Build Path(base path=w507, name or relative path=w505) -> (appended path=w504:path)
        n244 = Bundle By Name(cluster=w502, "Date FolderPath"=w504) -> (w503:T5)
      }
      frame "Compare Files" {
        # "would still be missing in/out of tol on tracking"
        n245 = Unbundle By Name(w526) -> ("RIOTempFolder"=w522:path)
        n246 = local read "IP 4"() -> (w527:u8)
        n247 = Format Into String(format string="%g.cal", w527) -> (resulting string=w525:string)  [unwired: 2 in, 1 out]
        n248 = Build Path(base path=w522, name or relative path=w525) -> (appended path=w529:path)
        n249 = Build Path(base path=w522, name or relative path="Setup.info") -> (appended path=w519:path)
        n250 = call "Simple CSV.vi"("Filepath In"=w529, "Mode"=enum16{"Read", "Write"}."Read") -> ("Data Out"=w524:string[][])  [unwired: 11 in, 2 out]
        n251 = call "Simple CSV.vi"("Filepath In"=w519, "Mode"=enum16{"Read", "Write"}."Read") -> ("Data Out"=w518:string[][])  [unwired: 11 in, 2 out]
        n252 = call "Parse RIO cal file.vi"("Data In"=w524) -> ()  [unwired: 10 in, 5 out]
        n253 = call "Parse Setup file.vi"("Data In"=w518) -> ()  [unwired: 8 in, 7 out]
      }
      frame "Read Data" {
        n254 = Unbundle By Name(w532) -> ("MaskReadings"=w531:bool)
        n255 = call "Machine Cal Data Engine (global).vi"("Mode"=T7."Read Data") -> ("Data Out"=w537:dbl[], "New Data"=w538:bool, "Connection"=w535:bool)  [unwired: 11 in, 1 out]
        n256 = case shown="True" w535 {
          tunnel: w538 -> [_ w550]
          tunnel: w537 -> [_ w549]
          tunnel: w532 -> [w544 w548]
          tunnel: [w544 w547] -> w536
          tunnel: w534 -> [w543 w546]
          tunnel: [w542 w546] -> w533
          tunnel: w531 -> [_ w545]
          frame False {
            n257 = Insert Into Array(array=w543, index=0, new element="Data Stream Lost" ("new element/subarray")) -> (w542:string[])
          }
          frame True {
            n258 = case shown="True" w545 {
              tunnel: w550 -> [_ w568]
              tunnel: w549 -> [w554 w567]
              tunnel: w548 -> [w556 w566]
              tunnel: [w555 w565] -> w547
              frame True {
                # "Clear readings from unselected ch.s"
                # "Cal/Ver ch.s\ndisplayed"
                # "All Channels\nin system"
                # "All Ch.s selected\nfor Cal/Ver"
                # "Masking all readings\n   allows finishing a cal"
                n259 = Unbundle By Name(w556) -> ("Read Array"=w559:bool[])
                n260 = for {
                  tunnel: w554 -> [_] mode=indexing
                  tunnel: [nan ("f")] -> w553 mode=indexing
                }
                n261 = for {
                  tunnel: w553 -> [w564] mode=indexing
                  tunnel: w559 -> [w563] mode=indexing
                  tunnel: [w564] -> w557 mode=indexing if=w563
                }
                n262 = Array Subset(array=w557, index=0, length=12) -> (w552:dbl[])
                n263 = Get Date/Time In Seconds() -> (seconds since 1Jan1904=w561:timestamp)
                n264 = To Double Precision Float(number=w561) -> (double precision float=w560:dbl)
                n265 = Bundle By Name(cluster=w556, "Data Timer"=w560, "Full Data"=w553, "Cal/Ver Data"=w557) -> (w555:T5)
                n266 = local write "Readings"(w552) -> ()
              }
              frame False {
                # "Continue as normal"
                n267 = case shown="True" w568 {
                  tunnel: w567 -> [_ w572]
                  tunnel: w566 -> [w570 w579]
                  tunnel: [w570 w580] -> w565
                  frame False {
                    # "Still have a connection\nbut no new data"
                    n268 = Wait (ms)(milliseconds to wait=u32 2) -> ()  [unwired: 1 out]
                  }
                  frame True {
                    # "Clear readings from unselected ch.s"
                    # "Cal/Ver ch.s\ndisplayed"
                    # "All Channels\nin system"
                    # "All Ch.s selected\nfor Cal/Ver"
                    n269 = Unbundle By Name(w579) -> ("Checkbox Array"=w574:bool[], "Channel Offset"=w577:i32, "Read Array"=w578:bool[])
                    n270 = for {
                      tunnel: w572 -> [w588] mode=indexing
                      tunnel: w578 -> [w587] mode=indexing
                      tunnel: [w588] -> w571 mode=indexing if=w587
                    }
                    n271 = Array Subset(array=w571, index=w577, length=12) -> (w575:dbl[])
                    n272 = for {
                      tunnel: w575 -> [w585] mode=indexing
                      tunnel: w574 -> [w586] mode=indexing
                      tunnel: [w584] -> w573 mode=indexing
                      n273 = Select(t=w585, s=w586, f=nan) -> (s? t:f=w584:dbl)
                    }
                    n274 = Get Date/Time In Seconds() -> (seconds since 1Jan1904=w582:timestamp)
                    n275 = To Double Precision Float(number=w582) -> (double precision float=w581:dbl)
                    n276 = Bundle By Name(cluster=w579, "Data Timer"=w581, "Full Data"=w572, "Cal/Ver Data"=w571) -> (w580:T5)
                    n277 = local write "Readings"(w573) -> ()
                  }
                }
              }
            }
          }
        }
      }
      frame "Take Reading" {
        n278 = Unbundle By Name(w610) -> ("CalState"=w606:string, "RoomTemp"=w593:dbl, "RelHumidity"=w592:dbl, "MasterReading"=w608:dbl, "CalChannelsStorage"=w597:string[][], "Read Array"=w599:bool[], "Full Data"=w600:dbl[], "CalChannelsDisplay"=w603:string[][], "Checkbox Array"=w604:bool[], "Cal/Ver Data"=w605:dbl[], "MasterCol"=w601:i32)
        n279 = Number To Fractional String(number=w593, precision (6)=i16 16) -> (F-format string=w591:string)  [unwired: 2 in]
        n280 = Number To Fractional String(number=w592, precision (6)=i16 16) -> (F-format string=w590:string)  [unwired: 2 in]
        n281 = Number To Fractional String(number=w608, precision (6)=i16 16) -> (F-format string=w598:string)  [unwired: 2 in]
        n282 = call "Take Reading.vi"("Data In"=w597, "RelHumidity"=w590, "RoomTemp"=w591, "Master Reading"=w598, "Write Array"=w599, "Data Readings"=w600, "MasterCol"=w601) -> ("Data Out"=w596:string[][])  [unwired: 8 in]
        n283 = call "Take Reading.vi"("Data In"=w603, "RelHumidity"=w590, "RoomTemp"=w591, "Master Reading"=w598, "Write Array"=w604, "Data Readings"=w605, "MasterCol"=w601) -> ("Data Out"=w602:string[][])  [unwired: 8 in]
        n284 = local write "Channels"(w602) -> ()
        n285 = case shown="\"Calibrate\", Default" w606 {
          tunnel: w610 -> [w612 w618 w622]
          tunnel: [w611 w617 w621] -> w609
          tunnel: w602 -> [w613 w616 w619]
          tunnel: w596 -> [w614 w615 w620]
          frame "As Found" {
            n286 = Bundle By Name(cluster=w612, "FoundChannelsStorage"=w614, "CalChannelsDisplay"=w613) -> (w611:T5)
          }
          frame "Calibrate", Default {
            n287 = Bundle By Name(cluster=w618, "CalChannelsStorage"=w615, "CalChannelsDisplay"=w616) -> (w617:T5)
          }
          frame "Verify" {
            n288 = Bundle By Name(cluster=w622, "VerChannelsStorage"=w620, "CalChannelsDisplay"=w619) -> (w621:T5)
          }
        }
      }
      frame "Finalize Files" {
        # "I think this case may be unneccessary\n\nwhenever programs read on Cal/Ver tab gets activated should establish connection\nand whenever it gets turned off (including automatically if leaving tab) stop connection\n\nso would just need to rename this and have it finish any file operations including dumping temp files"
      }
      frame "Create Date Folder" {
        n289 = Unbundle By Name(w642) -> ("ServerStorageFolder"=w650:path, "RIOprogram"=w626:string)
        n290 = local read "IP 1"() -> (w646:u8)
        n291 = local read "IP 2"() -> (w647:u8)
        n292 = local read "IP 3"() -> (w648:u8)
        n293 = local read "IP 4"() -> (w649:u8)
        n294 = Format Into String(format string="%g_%g_%g_%g", initial string="Storage\\", w646, w647, w648, w649) -> (resulting string=w644:string)  [unwired: 1 in, 1 out]
        n295 = Get Date/Time In Seconds() -> (seconds since 1Jan1904=w640:timestamp)
        n296 = Build Path(base path=w650, name or relative path=w644) -> (appended path=w638:path)
        n297 = call <vilib>:"Check if File or Folder Exists.vi"("path"=w638) -> ("error out"=w627:errorcluster, "file or folder exists?"=w637:bool, "dup path"=w636:path)  [unwired: 8 in]
        n298 = Format Date/Time String(time format string (%c)="%Y_%m_%d", seconds (now)=w640) -> (date/time string=w625:string)  [unwired: 1 in]
        n299 = case shown="False" w637 {
          tunnel: w636 -> [w660 w662]
          tunnel: w627 -> [w659 w661]
          tunnel: [w658 w662] -> w631
          tunnel: [w657 w661] -> w630
          frame False {
            n300 = Create Folder(path (use dialog)=w660, error in=w659) -> (created path=w658:path, error out=w657:errorcluster)  [unwired: 1 in, 1 out]
          }
          frame True {
          }
        }
        n301 = Concatenate Strings(w625, "_" ("string"), w626) -> (w624:string)
        n302 = Build Path(base path=w631, name or relative path=w624) -> (appended path=w632:path)
        n303 = call <vilib>:"Check if File or Folder Exists.vi"("error in (no error)"=w630, "path"=w632) -> ("error out"=w635:errorcluster, "file or folder exists?"=w633:bool, "dup path"=w634:path)  [unwired: 7 in]
        n304 = case shown="False" w633 {
          tunnel: w634 -> [w654 w656]
          tunnel: w635 -> [w653 w655]
          tunnel: [w652 w656] -> w629
          tunnel: [w651 w655] -> _
          frame False {
            n305 = Create Folder(path (use dialog)=w654, error in=w653) -> (created path=w652:path, error out=w651:errorcluster)  [unwired: 1 in, 1 out]
          }
          frame True {
          }
        }
        n306 = Bundle By Name(cluster=w642, "Date FolderPath"=w629) -> (w641:T5)
      }
      frame "Load Info/Channels" {
        w691 = 1 ("index")
        w700 = 1 ("index")
        w702 = 1 ("index")
        n307 = Unbundle By Name(w688) -> ("Date FolderPath"=w708:path)
        n308 = Build Path(base path=w708, name or relative path="All_Data.csv") -> (appended path=w706:path)
        n309 = call-poly <vilib>:"Read From Spreadsheet File.vi"("delimiter (\\t)"="," ("delimiter (\\t)"), "file path (dialog if empty)"=w706) -> ("all rows"=w696:string[][])  [unwired: 5 in, 4 out]
        n310 = Delete From Array(array=w696, length=21, index (row)=0) -> (deleted portion=w690:string[][], array with subset deleted=w681:string[][])  [unwired: 1 in]
        n311 = Index Array(array=w681, index (col)=0 ("disabled index (col)")) -> (element=w683:string[])  [unwired: 1 in]
        n312 = Search 1D Array(1D array=w683, element="Machine Specs - Unit:") -> (index of element=w669:i32)  [unwired: 1 in]
        n313 = Decrement(x=w669) -> (x-1=w670:i32)
        n314 = Increment(x=w669) -> (x+1=w668:i32)
        n315 = Array Subset(array=w690, index (row)=0 ("index"), length (row)=7 ("length"), index (col)=w702, length (col)=w702) -> (w701:string[][])
        n316 = Array Subset(array=w690, index (row)=7 ("index"), length (row)=8 ("length"), index (col)=w700, length (col)=w700) -> (w697:string[][])
        n317 = Array Subset(array=w690, index (row)=15 ("index"), length (row)=6 ("length"), index (col)=w691, length (col)=w691) -> (w689:string[][])
        n318 = Array Subset(array=w681, index (row)=1 ("index"), length (row)=w670, index (col)=0 ("index"), length (col)=5 ("length")) -> (w679:string[][])
        n319 = Search 1D Array(1D array=w683, element="Channel Desc. - Name:") -> (index of element=w666:i32)  [unwired: 1 in]
        n320 = Subtract(x=w666, y=w668) -> (x-y=w667:i32)
        n321 = Increment(x=w666) -> (x+1=w665:i32)
        n322 = Array Subset(array=w681, index (row)=w668, length (row)=w667, index (col)=0 ("index"), length (col)=8 ("length")) -> (w678:string[][])
        n323 = Search 1D Array(1D array=w683, element="Tracking - Name:") -> (index of element=w664:i32)  [unwired: 1 in]
        n324 = Subtract(x=w664, y=w665) -> (x-y=w663:i32)
        n325 = Array Subset(array=w681, index (row)=w665, length (row)=w663, index (col)=0 ("index"), length (col)=4 ("length")) -> (w677:string[][])
        n326 = Bundle By Name(cluster=w688, "Environment Details"=w701, "Instrument Identification"=w697, "Standards Used"=w679, "Calibration Details"=w689, "Machine Specifications:"=w678, "Channel Descriptions:"=w677) -> (w687:T5)
      }
      frame "Clear Info/Channels" {
        w710 = string[][] [] ("Instrument Identification")
        n327 = Bundle By Name(cluster=w714, "Environment Details"=string[][] [["TI Automotive"], ["Caro Test Center"], ["628 Columbia St."], ["Caro, MI 48723"], [""], [""], [""]], "Instrument Identification"=w710, "Standards Used"=w710, "Calibration Details"=w710, "Machine Specifications:"=w710, "Channel Descriptions:"=w710) -> (w713:T5)
      }
      frame "Load Select/Tracking" {
        n328 = Unbundle By Name(w733) -> ("Date FolderPath"=w739:path)
        n329 = Build Path(base path=w739, name or relative path="All_Data.csv") -> (appended path=w737:path)
        n330 = call-poly <vilib>:"Read From Spreadsheet File.vi"("delimiter (\\t)"="," ("delimiter (\\t)"), "file path (dialog if empty)"=w737) -> ("all rows"=w715:string[][])  [unwired: 5 in, 4 out]
        n331 = Index Array(array=w715, index (col)=0 ("disabled index (col)")) -> (element=w720:string[])  [unwired: 1 in]
        n332 = Search 1D Array(1D array=w720, element="Tracking - Name:") -> (index of element=w729:i32)  [unwired: 1 in]
        n333 = Increment(x=w729) -> (x+1=w727:i32)
        n334 = Array Size(array=w720) -> (size(s)=w718:i32)
        n335 = Search 1D Array(1D array=w720, element="Channels - Channel:") -> (index of element=w717:i32)  [unwired: 1 in]
        n336 = Increment(x=w717) -> (x+1=w716:i32)
        n337 = Subtract(x=w717, y=w727) -> (x-y=w726:i32)
        n338 = Subtract(x=w718, y=w716) -> (x-y=w719:i32)
        n339 = Array Subset(array=w715, index (row)=w727, length (row)=w726, index (col)=0 ("index"), length (col)=7 ("length")) -> (w725:string[][])
        n340 = Array Subset(array=w715, index (row)=w716, length (row)=w719, index (col)=0 ("index"), length (col)=11 ("length")) -> (w721:string[][])
        n341 = Bundle By Name(cluster=w733, "Tracking"=w725, "CalChannelsStorage"=w721) -> (w732:T5)
      }
      frame "Clear Select/Tracking" {
      }
      frame "Save System Information" {
        # "I can already open a seperate incidence of Excel\nbut can it be kept hidden?\nif so I should just keep the file open"
        n342 = Unbundle By Name(w740) -> ()  [unwired: 7 out]
        n343 = call "Excel___Write System Information.vi"() -> ()  [unwired: 12 in]
      }
      frame "Display Info Tab" {
        n344 = Unbundle By Name(w742) -> ("Environment Details"=w746:string[][], "Instrument Identification"=w745:string[][], "Standards Used"=w744:string[][], "Calibration Details"=w743:string[][])
        n345 = local write "Environment Details"(w746) -> ()
        n346 = local write "Instrument Identification"(w745) -> ()
        n347 = local write "Standards Used"(w744) -> ()
        n348 = local write "Calibration Details"(w743) -> ()
      }
      frame "Display Chan Setup Tab" {
        n349 = Unbundle By Name(w748) -> ("Machine Specifications:"=w750:string[][], "Channel Descriptions:"=w749:string[][])
        n350 = local write "Machine Specifications:"(w750) -> ()
        n351 = local write "Channel Descriptions:"(w749) -> ()
      }
      frame "Display Selection Tab" {
        w756 = i32[] [] ("TrackingRowsSel")
        n352 = Unbundle By Name(w760) -> ("CalChannelsStorage"=w751:string[][], "Machine Specifications:"=w768:string[][], "TrackingTableColors"=w754:i32[][])
        n353 = Index Array(array=w768, index (col)=1 ("disabled index (col)")) -> (element=w766:string[])  [unwired: 1 in]
        n354 = Sort 1D Array(array=w766) -> (sorted array=w765:string[])
        n355 = call "Color Tracking Table.vi"("Mode"=enum16{"Select", "Track"}."Track", "TrackingTableColors"=w754) -> ()  [unwired: 10 in]
        n356 = Insert Into Array(array=w765, index=0, new element="") -> (w763:string[])
        n357 = local write "Tracking"(w751) -> ()
        n358 = property on="Select Units:" class="Enum (strict)"("Strings []"=w763, "Value"=0) -> ()  [unwired: 2 in, 2 out]
        n359 = local write "Channels Selected:"(0 ("Channels Selected:")) -> ()
        n360 = property on="pb.Cal/Ver_Forward" class="Bool"("DisabledEnum"=T6."Disabled and Grayed Out" ("Disabled")) -> ()  [unwired: 2 in, 2 out]
        n361 = Bundle By Name(cluster=w760, "TrackingRowsSel"=w756) -> (w759:T5)
        n362 = call "Color Tracking Table.vi"("Mode"=enum16{"Select", "Track"}."Select", "TrackingRowsSelected"=w756) -> ()  [unwired: 10 in]
      }
      frame "Display Cal/Ver Tab" {
        # "Meant for scrolling\nto top of data"
        n363 = Unbundle By Name(w794) -> ("CalChannelsStorage"=w792:string[][], "TrackingRowsSel"=w791:i32[], "Machine Specifications:"=w776:string[][])
        n364 = local read "Select Units:"() -> (w777:enum16{""})
        n365 = property on="Select Units:" class="Enum (strict)"() -> ("Strings []"=w778:string[])  [unwired: 2 in, 2 out]
        n366 = for {
          shift-right: [w805] -> _
          shift-left: w792 -> [w805]
          tunnel: w791 -> [w804] mode=indexing
          tunnel: [w800] -> w784 mode=concatenating
          n367 = Array Subset(array=w805, index (row)=w804, length (row)=1 ("length"), index (col)=4 ("index"), length (col)=1 ("length")) -> (w800:string[][])
        }
        n368 = Index Array(array=w776, index (col) #1=0 ("disabled index (col)"), index (col) #2=1 ("index (col)")) -> (element #1=w771:string[], element #2=w773:string[])  [unwired: 2 in]
        n369 = Index Array(array=w778, index=w777) -> (element=w772:string)
        "Unit Abbreviation" <- w772
        n370 = Search 1D Array(1D array=w773, element=w772) -> (index of element=w770:i32)  [unwired: 1 in]
        n371 = Index Array(array=w771, index=w770) -> (element=→"Units":string)
        n372 = Greater?(x="Channels Selected:", y=12) -> (0:w795:bool)
        n373 = Array Size(array=w784) -> (size(s)=w783:i32[])
        n374 = Index Array(array=w783, index=0) -> (element=w781:i32)
        n375 = Select(t=u32 804 ("Size:Width"), s=w795, f=u32 787 ("Size:Width")) -> (s? t:f=w798:u32)
        n376 = local write "Channels"(w784) -> ()
        n377 = property on="Readings" class="Arr (strict)"("Number of Rows"="Channels Selected:") -> ()  [unwired: 2 in, 2 out]
        n378 = property on="Channels" class="Tbl (strict)"("Width"=w798, "Vert Scrollbar"=w795) -> ()  [unwired: 2 in, 2 out]
        n379 = Initialize Array(FALSE, w781) -> (w780:bool[])
        n380 = Bundle By Name(cluster=w794, "Scroll Check"=w795, "Checkbox Array"=w780, "CalChannelsDisplay"=w784) -> (w793:T5)
        n381 = property on="Channels" class="Tbl (strict)"("Selection Start"=T9 {"Row"=0, "Column"=0} ("Active Cell:Active Cell")) -> ()  [unwired: 2 in, 2 out]
        n382 = call "Checkbox Display.vi"("Starting Row"=0, "Checkbox Array"=bool[] [FALSE, FALSE, FALSE, FALSE, FALSE, FALSE, FALSE, FALSE, FALSE, FALSE, FALSE, FALSE]) -> ()  [unwired: 10 in]
      }
      frame "Scroll Channels" {
        w811 = 12 ("length")
        n383 = Unbundle By Name(w816) -> ("Checkbox Array"=w812:bool[])
        n384 = property on="Channels" class="Tbl (strict)"() -> ("Selection Start"=w813:T9)  [unwired: 2 in, 2 out]
        n385 = Unbundle(w813) -> ("Row"=w808:i32)  [unwired: 1 out]
        n386 = Array Size(array=w812) -> (size(s)=w809:i32)
        n387 = Add(x=w811, y=w808) -> (x+y=w810:i32)
        n388 = Array Subset(array=w812, index=w808, length=w811) -> (w807:bool[])
        n389 = Subtract(x=w810, y=w809) -> (x-y=w806:i32)
        n390 = Bundle By Name(cluster=w816, "Channel Offset"=w808) -> (w815:T5)
        n391 = call "Checkbox Display.vi"("Starting Row"=w806, "Checkbox Array"=w807) -> ()  [unwired: 10 in]
      }
      frame "Return to Login" {
        w820 = u16 0 items=["", "Start Calibration", "Continue Calibration", "System Initialization", "System Closeout"] ("Action to Perform")
        w821 = u8 0 ("IP 1")
        n392 = local write "Tab.Screen"(T1."Login" ("Tab.Screen")) -> ()
        n393 = local write "IP 1"(w821) -> ()
        n394 = local write "IP 2"(w821) -> ()
        n395 = local write "IP 3"(w821) -> ()
        n396 = local write "IP 4"(w821) -> ()
        n397 = local write "Action to Perform"(w820) -> ()
        n398 = property on="pb.sys_connect" class="Bool"("DisabledEnum"=T6."Disabled and Grayed Out" ("Disabled")) -> ()  [unwired: 2 in, 2 out]
      }
      frame "Freeze Screen", "Thaw Screen" {
        n399 = control-ref of="This VI"() -> (w831:refnum<vi>)
        n400 = String Subset(string=w829, length (rest)=0 ("length (rest)")) -> (substring=w827:string)  [unwired: 1 in]
        n401 = property class="VI"(reference=w831) -> ("Panel"=w830:refnum<vi>)  [unwired: 1 in, 2 out]
        n402 = Not Equal?(x="Thaw", y=w827) -> (x != y?=w825:bool)
        n403 = property class="Pnl"(reference=w830, "DeferPanUpdts"=w825) -> ()  [unwired: 1 in, 2 out]
      }
      frame "Set Cursor Busy" {
        n404 = call <vilib>:"Set Busy.vi"() -> ()  [unwired: 10 in, 2 out]
      }
      frame "Unset Cursor Busy" {
        n405 = call <vilib>:"Unset Busy.vi"() -> ()  [unwired: 11 in, 1 out]
      }
      frame "System Not Found", "System Not Registered" {
        n406 = String Subset(string=w844, offset (0)=11, length (rest)=5 ("length (rest)")) -> (substring=w841:string)
        n407 = Equal?(x=w841, y="Found") -> (x = y?=w837:bool)
        n408 = Select(t=enum32{"Registration", "Connection"}."Connection" ("Connection Error"), s=w837, f=enum32{"Registration", "Connection"}."Registration" ("Connection Error")) -> (s? t:f=w836:enum32{"Registration", "Connection"})
        n409 = local write "Connection Error"(w836) -> ()
        n410 = for {
          tunnel: bool[] [TRUE, FALSE, TRUE, FALSE] -> [w851] mode=indexing
          tunnel: u32[] [300, 300, 300, 1] -> [w849] mode=indexing
          tunnel: w836 -> [_]
          n411 = flat-sequence {
            tunnel: w851 -> [w853]
            tunnel: [w852] -> w850
            tunnel: w849 -> [w852]
            tunnel: w850 -> [w854]
            frame #0 {
              n412 = property on="Connection Error" class="TabCtl (strict)"("Visible"=w853) -> ()  [unwired: 2 in, 2 out]
            }
            frame #1 {
              n413 = Wait (ms)(milliseconds to wait=w854) -> ()  [unwired: 1 out]
            }
          }
        }
      }
      frame "RIO Import Error" {
        w855 = T1."Login" ("Tab.Screen")
        w860 = T2."RIO Import" ("Connection Error")
        n414 = local write "Connection Error"(w860) -> ()
        n415 = local write "Tab.Screen"(w855) -> ()
        n416 = for {
          tunnel: bool[] [TRUE, FALSE, TRUE, FALSE] -> [w866] mode=indexing
          tunnel: u32[] [300, 300, 300, 1] -> [w864] mode=indexing
          tunnel: w860 -> [_]
          tunnel: w855 -> [_]
          n417 = flat-sequence {
            tunnel: w866 -> [w868]
            tunnel: [w867] -> w865
            tunnel: w864 -> [w867]
            tunnel: w865 -> [w869]
            frame #0 {
              n418 = property on="Connection Error" class="TabCtl (strict)"("Visible"=w868) -> ()  [unwired: 2 in, 2 out]
            }
            frame #1 {
              n419 = Wait (ms)(milliseconds to wait=w869) -> ()  [unwired: 1 out]
            }
          }
        }
        n420 = Insert Into Array(array=w857, index=0, new element=string[] ["Unset Cursor Busy"]) -> (w856:string[])
      }
      frame "Unused" {
      }
    }
  }
  n421 = flat-sequence {
    tunnel: w14 -> [w872]
    frame #0 {
      n422 = Wait on Occurrence(2:w872) -> ()  [unwired: 2 in, 1 out]
    }
    frame #1 {
      n423 = call "Machine Cal Data Engine.vi"() -> ()  [unwired: 12 in]
    }
  }
  n424 = disable-structure shown="Disabled" {
    frame Disabled {
      n425 = call "Table Control_2D.vi"() -> ()  [unwired: 14 in, 2 out]
    }
    frame Enabled {
    }
  }
  n426 = property on="pb.Cal/Ver_Forward" class="Bool" props=["BoolText", "Text"]() -> ()  [unwired: 3 in, 2 out]
  n427 = disable-structure shown="Disabled" {
    frame Disabled {
      n428 = call <vilib>:"Mean PtByPt.vi"() -> ()  [unwired: 4 in, 2 out]
      n429 = call "D2A_5V.vi"() -> ()  [unwired: 15 in, 1 out]
    }
    frame Enabled {
    }
  }
  n430 = disable-structure shown="Disabled" {
    frame Disabled {
      n431 = call "Open Office File.vi"() -> ()  [unwired: 11 in, 1 out]
    }
    frame Enabled {
    }
  }
  n432 = call <vilib>:"General Polynomial Fit Coefficients.vi"("polynomial order"=4) -> ()  [unwired: 13 in, 2 out]
  n433 = Format Date/Time String(time format string (%c)="%d%b%y %I:%M:%S %p") -> (date/time string=w5:string)  [unwired: 2 in]
  n434 = To Upper Case(1:w5) -> ()  [unwired: 1 out]
  n435 = disable-structure shown="Disabled" {
    frame Disabled {
      n436 = call "Calc Dev (DAQ Rack).vi"() -> ()  [unwired: 19 in, 1 out]
    }
    frame Enabled {
    }
  }
  n437 = disable-structure shown="Disabled" {
    frame Disabled {
      # "Verify Table\nEdit Position\nproperty"
      # "Verify table"
      # "Auto boolean (for auto verify routine)"
      # "Ver Reading (reading with coefficients applied)"
      # "ms u32"
      n438 = Unbundle() -> (w893:T9, "Row"=w891)  [unwired: 1 out]
      n439 = Greater Or Equal To 0?(x=w891) -> (x >= 0?=w892:bool)
      n440 = Index Array(index (row)=w891, index (col)=0 ("disabled index (col)")) -> (array=w880:string[][], element=w883)
      n441 = case shown="True" w892 {
        tunnel: w891 -> [_ w895]
        frame False {
        }
        frame True {
          # "Row\nIndex\nI32"
        }
      }
      n442 = Fract/Exp String To Number(string=w883) -> (number=w875:dbl)  [unwired: 3 in, 1 out]
      n443 = Increment() -> (x=w873:dbl, x+1=w884:dbl)
      n444 = Increment(x=w875) -> (x+1=w885:dbl)
      n445 = Subtract(x=w884, y=w885) -> (x-y=w876:dbl)
      n446 = Divide(x=w876, y=w884) -> (x/y=w889:dbl)
      n447 = Empty String/Path?(string/path=w883) -> (empty?=w878:bool)
      n448 = Absolute Value(x=w889) -> (abs(x)=w874:dbl)
      n449 = Not(x=w878) -> (.not. x?=w886:bool)
      n450 = Less?(x=w874, y=0.1) -> (x < y?=w887:bool)
      n451 = Compound Arithmetic op=AND(w887, w886) -> (w882:bool, w879:bool)
      n452 = call "Reading Delay.vi"("In Range"=w882) -> ("Take Reading"=w877:bool, "Delay"=w881:u32)  [unwired: 9 in]
      n453 = case shown="True" w877 {
        selector: w877 -> [_ w894]
        frame False {
        }
        frame True {
          # "Verify Read\nVal(Sgnl)"
        }
      }
    }
    frame Enabled {
    }
  }
  n454 = disable-structure shown="Disabled" {
    disable-tunnel: _ -> [w897 _]
    disable-tunnel: _ -> [w896 _]
    frame Disabled {
      n455 = case shown="True" w896 {
        tunnel: w897 -> [_ w898]
        frame False {
        }
        frame True {
          w899 = FALSE
          # "ID"
          n456 = Format Into String(format string="ni.var.psp://10.30.189.%s/Streaming Control/StreamCalibrated", w898) -> (resulting string=w905:string, error out=w906:errorcluster)  [unwired: 2 in]
          n457 = shared-variable-open(w905, w906, w899) -> (w900:refnum<k21>, w903:errorcluster)  [unwired: 1 in]
          n458 = shared-variable-write(w900, w903, w899) -> (w901:refnum<k21>, w902:errorcluster)
          n459 = Close Variable Connection(8:w902, 11:w901) -> ()  [unwired: 1 out]
        }
      }
    }
    frame Enabled {
    }
  }
